vi "Taste Awful.vi"(11 "Array":i32[][](array[numeric])) -> (3 "logical AND":bool)   [LabVIEW 2014]
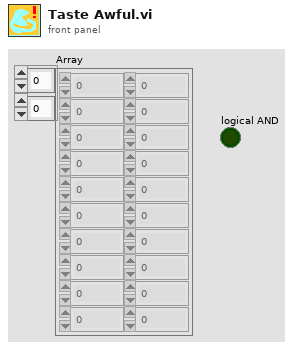
[diagram p1: front panel]
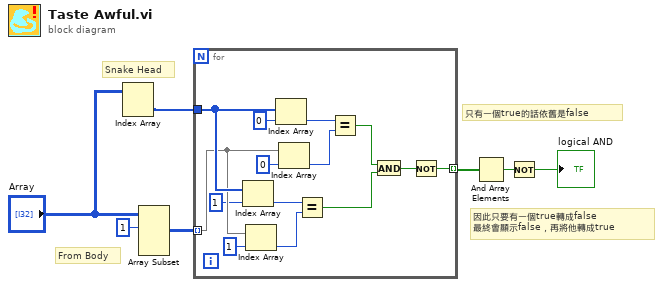
[diagram p0: block diagram]
diagram:
  # "因此只要有一個true轉成false\n最終會顯示false，再將他轉成true"
  # "只有一個true的話依舊是false"
  # "From Body"
  # "Snake Head"
  n1 = Index Array(array="Array") -> (element=w4:i32[])  [unwired: 2 in]
  n2 = Array Subset(array="Array", index (row)=1 ("index")) -> (w6:i32[][])  [unwired: 3 in]
  n3 = for {
    tunnel: w4 -> [w15]
    tunnel: w6 -> [w14] mode=indexing
    tunnel: [w8] -> w7 mode=indexing
    n4 = Index Array(array=w15, index=1) -> (element=w17:i32)
    n5 = Index Array(array=w14, index=1) -> (element=w16:i32)
    n6 = Index Array(array=w15, index=0) -> (element=w19:i32)
    n7 = Index Array(array=w14, index=0) -> (element=w18:i32)
    n8 = Equal?(x=w17, y=w16) -> (x = y?=w10:bool)
    n9 = Equal?(x=w19, y=w18) -> (x = y?=w11:bool)
    n10 = And(x=w11, y=w10) -> (x .and. y?=w9:bool)
    n11 = Not(x=w9) -> (.not. x?=w8:bool)
  }
  n12 = And Array Elements(Boolean array=w7) -> (logical AND=w2:bool)
  n13 = Not(x=w2) -> (.not. x?=→"logical AND":bool)
